vi "setAO_Amp.vi"(8 "error in (no error)":errorcluster, 9 "Amplitude (V)":dbl, 10 "AO Channel":i32=1 min=1 max=16, 11 "Instrument.Lockin in":refnum<class "Instrument.Lockin.lvclass">) -> (0 "error out":errorcluster, 3 "Instrument.Lockin out":refnum<class "Instrument.Lockin.lvclass">)   [LabVIEW 2019, in "Instrument.Lockin.lvlib" / "Instrument.Lockin.lvclass"]
doc: "API to configure an AO Amplitude.\n\nSpecify which channel you want to change and the value you want to set.\n\nIf address=\"\", this API reads from localhost\nIf address is remote lockin, you need to add this computer to allowed whitelist on the lockin computer you are trying to access."
uses:
  Instrument.Lockin.lvclass
  <userlib>/LevyLab/Instrument Framework/Instrument Types/Lockin/Instrument.LockinAPI.lvclass
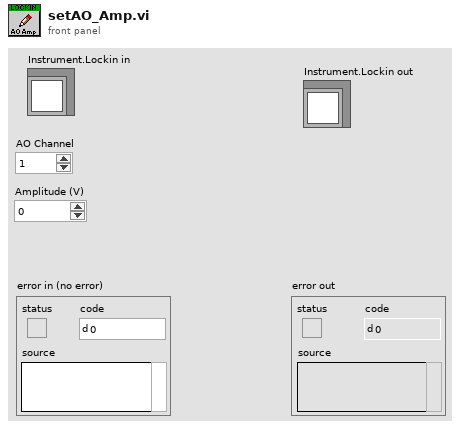
[diagram p1: front panel]
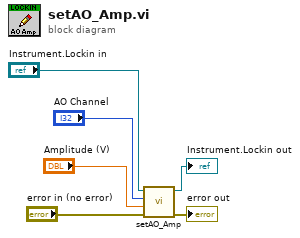
[diagram p0: block diagram]
diagram:
  n1 = call-parent "setAO_Amp.vi"("error in (no error)"="error in (no error)", "Amplitude (V)"="Amplitude (V)", "AO Channel"="AO Channel", "Instrument.LockinAPI in"="Instrument.Lockin in") -> ("error out"=→"error out":errorcluster, "Instrument.LockinAPI out"=→"Instrument.Lockin out":refnum<class "Instrument.Lockin.lvclass">)  [unwired: 6 in]
